vi "General Config.vi"(8 "error In":errorcluster, 10 "IOList":T2, 11 "reference":refnum<vi>) -> (0 "error out":errorcluster, 3 "Out reference":refnum<vi>)   [LabVIEW 2015]
uses:
  Control Button/Exit.ctl
  Control Button/Daq.ctl
  Control Button/Scanner config.ctl
  Control Button/Program Seq.ctl
  Control Button/cali.ctl
  Control Button/shift change.ctl
  Control Button/User mgt.ctl
  Control Button/model create.ctl
  Galobal variable_TI.vi
panel:
  in  "Image Setting":bool
  out "User Name 4":string
  in  "Load Cell Setting":bool
  out "User Name 3":string
  in  "Model Create":T1
  in  "User Mgt":T3
  out "User Name 2":string
  in  "Shift":T4
  in  "Calibration":T5
  in  "IO List Update":bool
  out "error out 2":errorcluster
  in  "error in (no error)":errorcluster
  in  "Program Seq":T6
  in  "Scanner config":T7
  in  "DAQ Config":T8
  out "User Name":string
  in  "Exit":T9
  out "String":string
  out "appended path":path
  in  "Ring":u16(ring)
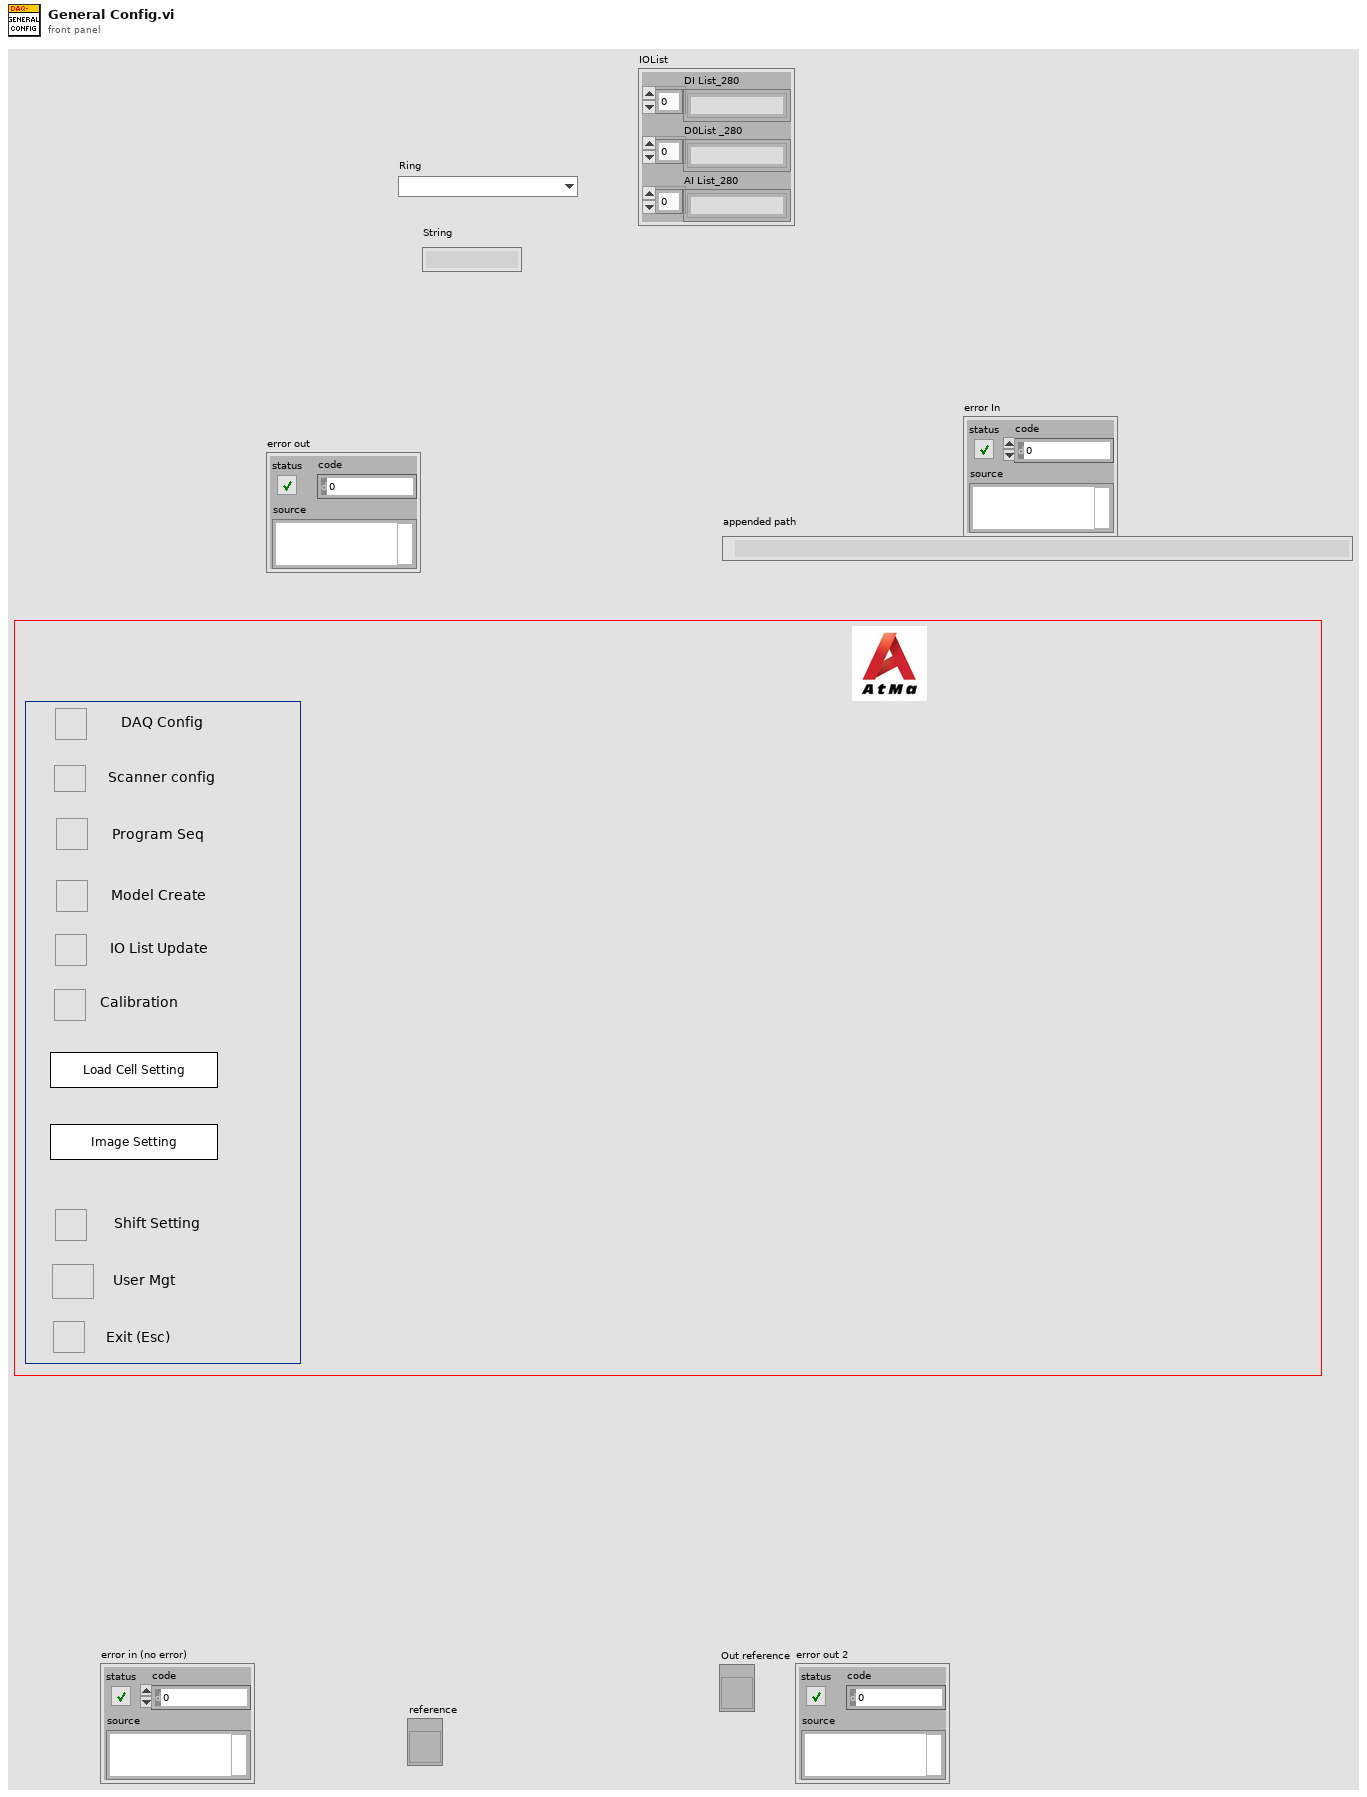
[diagram p1: front panel]
types:
  T1 = typedef "model create.ctl" = bool
  T2 = cluster{"DI List_280":string[], "D0List _280":string[], "AI List_280":string[]}
  T3 = typedef "User mgt.ctl" = bool
  T4 = typedef "shift change.ctl" = bool
  T5 = typedef "cali.ctl" = bool
  T6 = typedef "Program Seq.ctl" = bool
  T7 = typedef "Scanner config.ctl" = bool
  T8 = typedef "Daq.ctl" = bool
  T9 = typedef "Exit.ctl" = bool
  T10 = enum32{"Invalid", "Standard", "Closed", "Hidden", "Minimized", "Maximized"}
  T11 = cluster{"XInput":dbl[], "Y New Value":dbl[], "Avg point":i16}[]
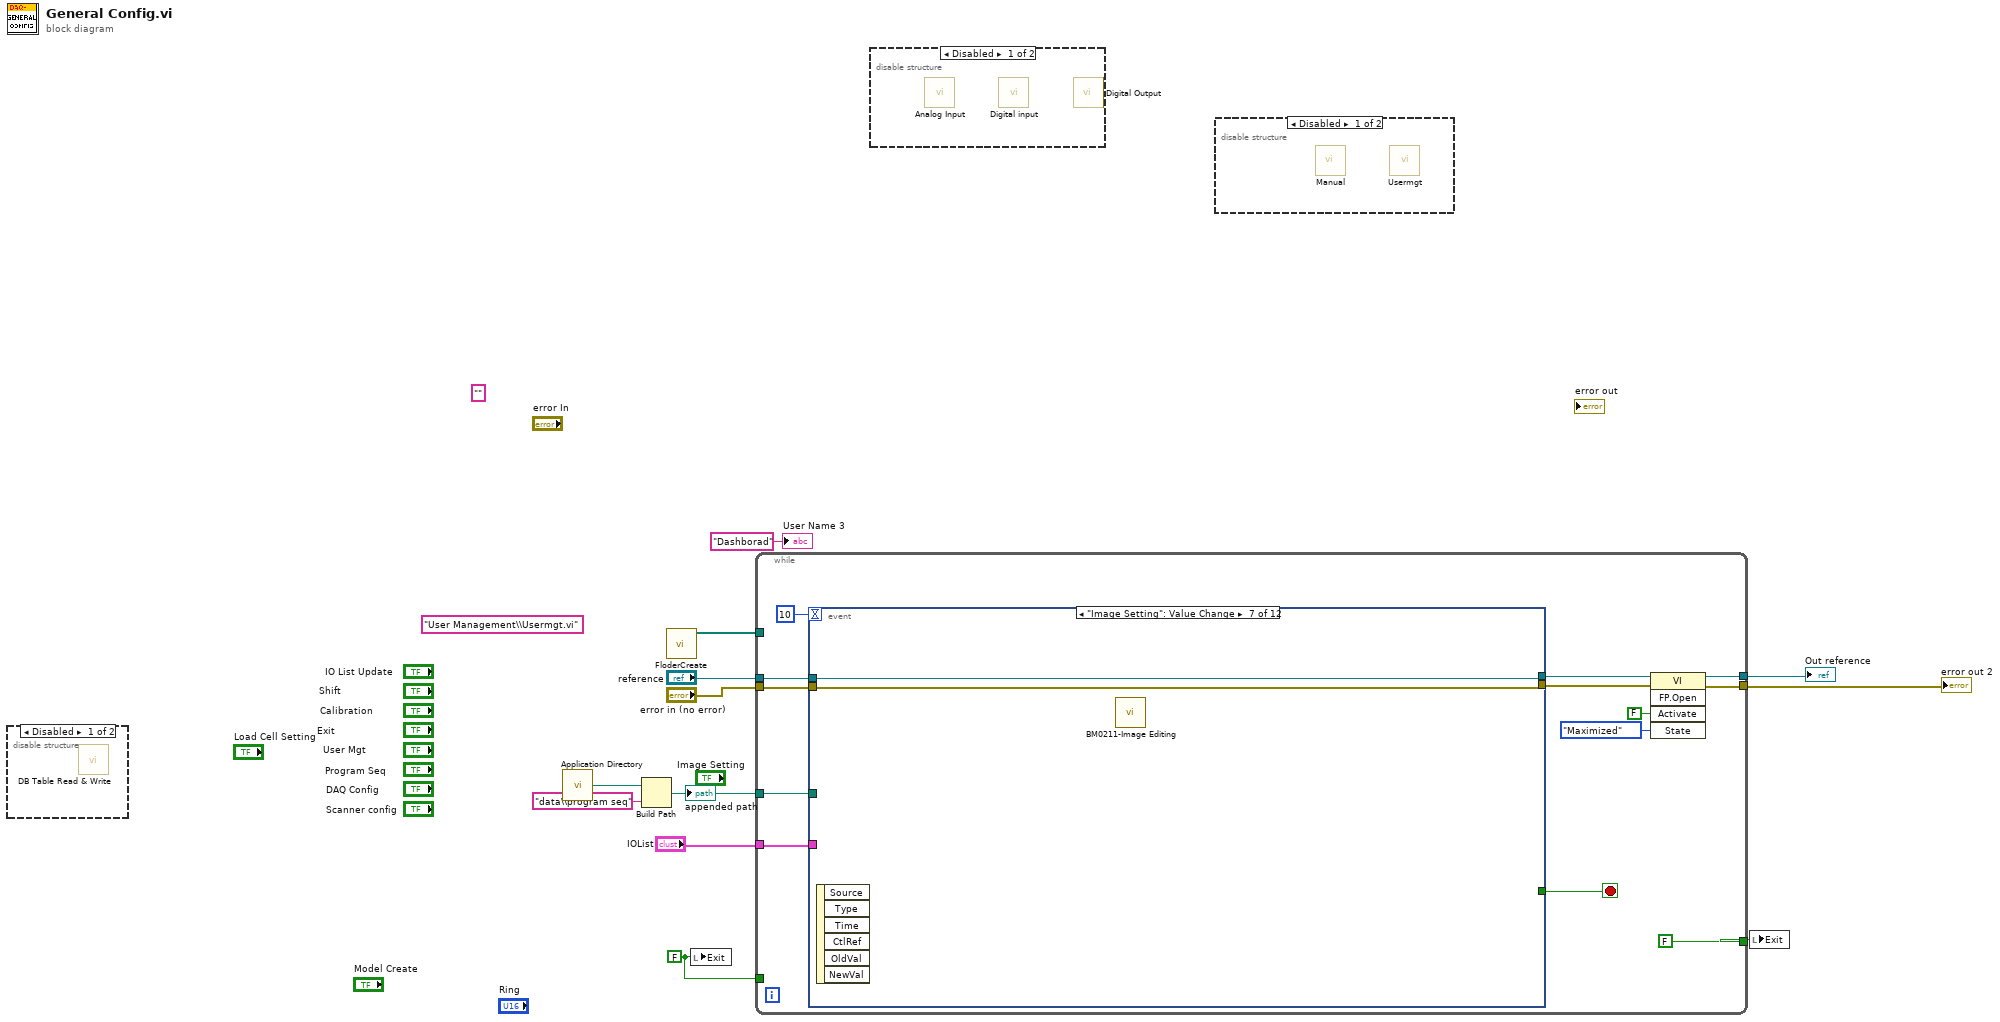
[diagram p0: block diagram]
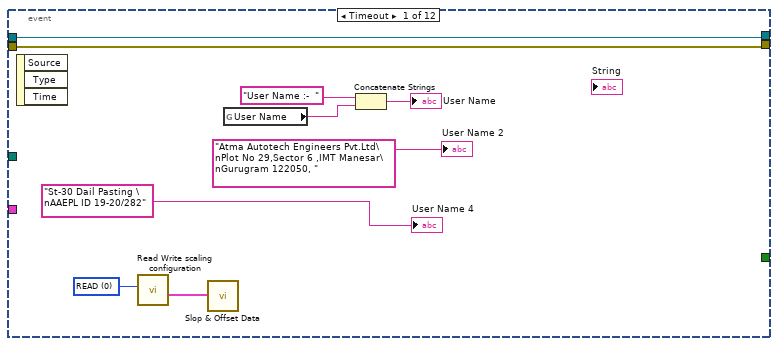
[diagram p5: hidden frame]
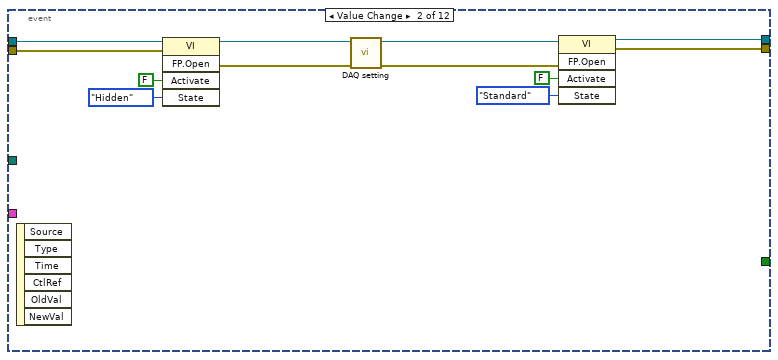
[diagram p6: hidden frame]
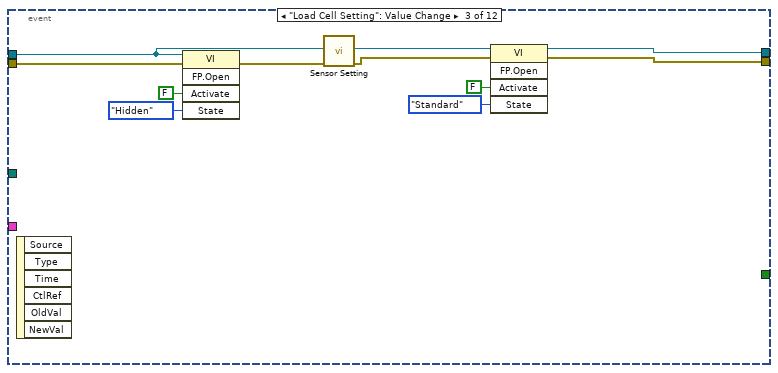
[diagram p7: hidden frame]
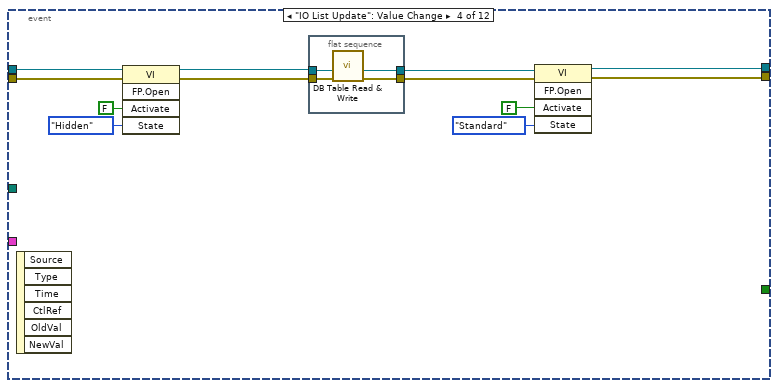
[diagram p8: hidden frame]
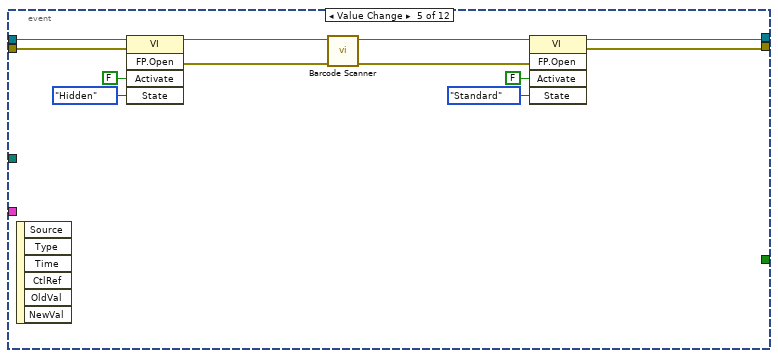
[diagram p9: hidden frame]
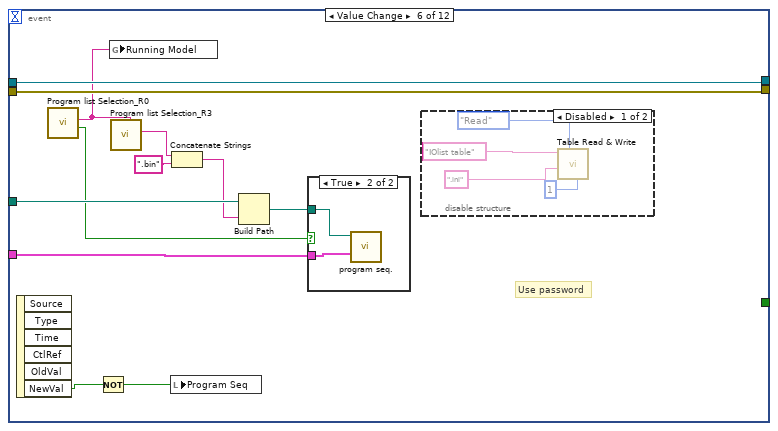
[diagram p10: hidden frame]
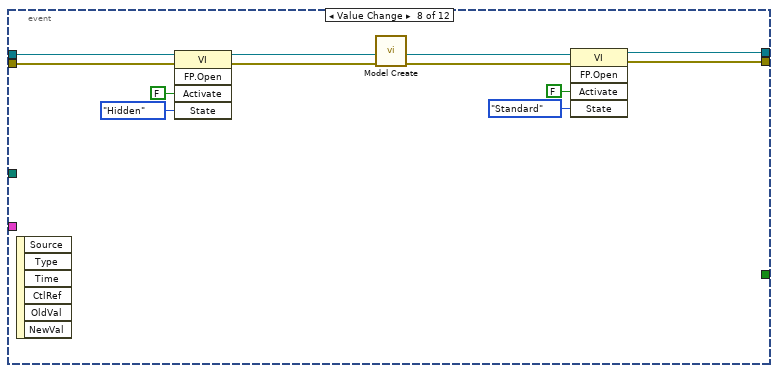
[diagram p13: hidden frame]
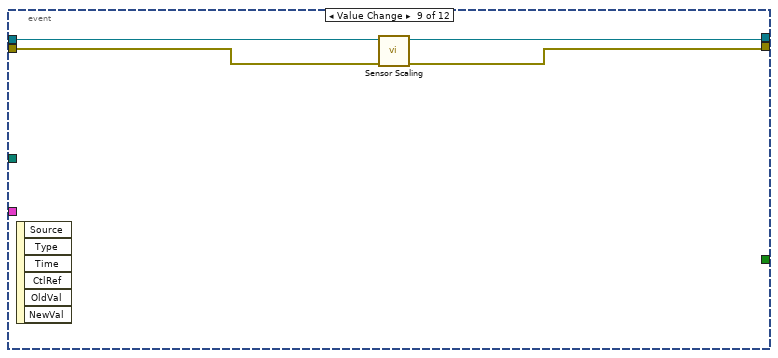
[diagram p14: hidden frame]
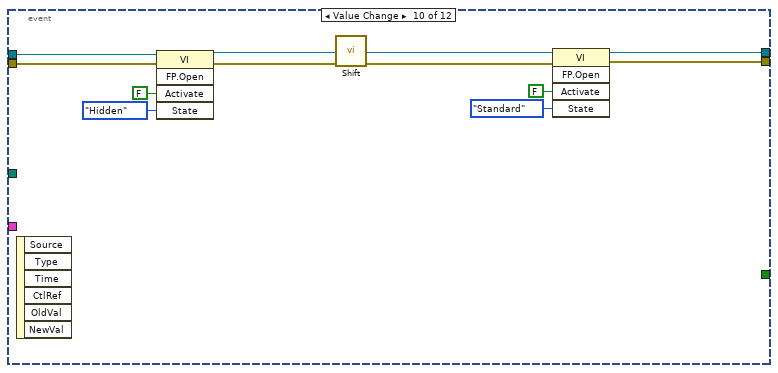
[diagram p15: hidden frame]
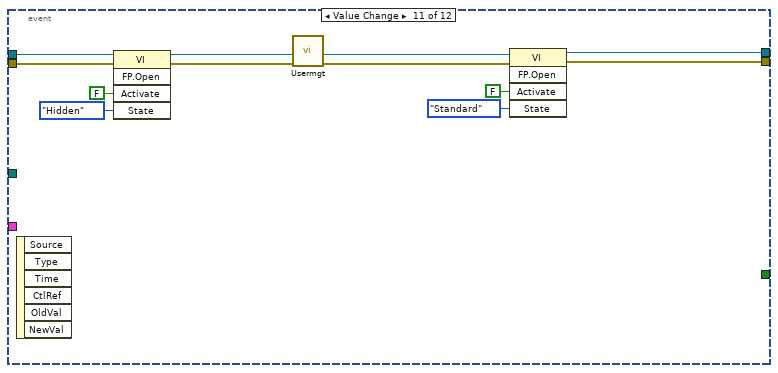
[diagram p16: hidden frame]
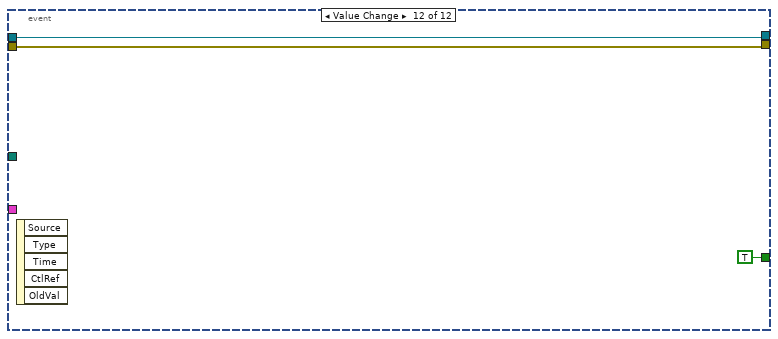
[diagram p17: hidden frame]
diagram:
  w9 = T9 FALSE ("Exit")
  (unwired) "User Management\\Usermgt.vi" ("name or relative path")
  (unwired) ""
  n1 = disable-structure shown="Disabled" {
    frame Disabled {
      n2 = call "DB Table Read & Write.vi"() -> ()  [unwired: 10 in, 2 out]
    }
    frame Enabled {
    }
  }
  n3 = call <vilib>:"Application Directory.vi"() -> ("Application Directory"=w5:path)
  n4 = Build Path(base path=w5, name or relative path="data\\program seq") -> (appended path=w2:path)
  "appended path" <- w2
  n5 = call "FloderCreate.vi"() -> ("File Path"=w6:path[])  [unwired: 11 in]
  n6 = local write "Exit"(w9) -> ()
  n7 = while {
    tunnel: w2 -> [w13]
    tunnel: "reference" -> [w23]
    tunnel: "error in (no error)" -> [w22]
    tunnel: [w17] -> w11
    tunnel: [w16] -> w10
    tunnel: w9 -> [_]
    tunnel: [T9 FALSE ("Exit")] -> w8
    tunnel: w6 -> [_]
    tunnel: "IOList" -> [w14]
    stop <- w24 stop-if-true
    n8 = event shown="[6] \"Image Setting\": Value Change" {
      selector: _ -> [_ _ _ _ _ _ _ _ _ _ _ _]
      dyn-events: _ -> [_ _ _ _ _ _ _ _ _ _ _ _]
      timeout: 10 -> [_ _ _ _ _ _ _ _ _ _ _ _]
      tunnel: [_ _ _ _ _ _ _ _ _ _ _ TRUE ("Exit")] -> w24
      tunnel: w23 -> [w31 w38 w48 w60 w82 w96 w104 w111 w118 w126 w135 w143]
      tunnel: w22 -> [w30 w37 w50 w59 w81 w95 w103 w110 w117 w124 w133 w142]
      tunnel: [w31 w36 w47 w67 w74 w96 w104 w106 w118 w125 w134 w143] -> w19
      tunnel: [w30 w35 w49 w66 w73 w95 w103 w105 w116 w123 w132 w142] -> w18
      tunnel: w14 -> [_ _ _ _ _ w94 _ _ _ _ _ _]
      tunnel: w13 -> [_ _ _ _ _ w93 _ _ _ _ _ _]
      event Timeout {
        w29 = u16 0 items=["READ", "WRITE"] ("Read/Write")
        n9 = event-data() -> ()  [unwired: 1 in, 3 out]
        n10 = call "Read Write scaling configuration.vi"("Read/Write"=w29) -> ("Output"=w28:T11)  [unwired: 4 in, 2 out]
        n11 = call "Slop & Offset Data.vi"("Input"=w28) -> ()  [unwired: 10 in, 1 out]
        n12 = global read "Galobal variable_TI.vi" "User Name"() -> (w34:string)
        n13 = Concatenate Strings("User Name :-  " ("string"), w34) -> (→"User Name":string)
        "User Name 2" <- "Atma Autotech Engineers Pvt.Ltd\nPlot No 29,Sector 6 ,IMT Manesar\nGurugram 122050, " ("string")
        "User Name 4" <- "St-30 Dail Pasting \nAAEPL ID 19-20/282" ("string")
      }
      event Value Change {
        n14 = event-data() -> ()  [unwired: 1 in, 6 out]
        n15 = invoke class="VI" method="FP.Open"(reference=w38, error in=w37, "Activate"=FALSE ("Activate?"), "State"=T10."Hidden") -> (reference out=w44:refnum<vi>, error out=w43:errorcluster)  [unwired: 1 in, 3 out]
        n16 = call "DAQ setting.vi"("error in (no error)"=w43, "vi reference"=w44) -> ("error Out"=w39:errorcluster, "Out reference"=w40:refnum<vi>)  [unwired: 8 in]
        n17 = invoke class="VI" method="FP.Open"(reference=w40, error in=w39, "Activate"=FALSE ("Activate?"), "State"=T10."Standard") -> (reference out=w36:refnum<vi>, error out=w35:errorcluster)  [unwired: 1 in, 3 out]
      }
      event "Load Cell Setting": Value Change {
        n18 = event-data() -> ()  [unwired: 1 in, 6 out]
        n19 = invoke class="VI" method="FP.Open"(reference=w48, error in=w50, "Activate"=FALSE ("Activate?"), "State"=T10."Hidden") -> (error out=w54:errorcluster)  [unwired: 1 in, 4 out]
        n20 = call "Sensor Setting.vi"("error in"=w54) -> ("error  out"=w51:errorcluster)  [unwired: 10 in]
        n21 = invoke class="VI" method="FP.Open"(reference=w48, error in=w51, "Activate"=FALSE ("Activate?"), "State"=T10."Standard") -> (reference out=w47:refnum<vi>, error out=w49:errorcluster)  [unwired: 1 in, 3 out]
      }
      event "IO List Update": Value Change {
        n22 = event-data() -> ()  [unwired: 1 in, 6 out]
        n23 = invoke class="VI" method="FP.Open"(reference=w60, error in=w59, "Activate"=FALSE ("Activate?"), "State"=T10."Hidden") -> (reference out=w58:refnum<vi>, error out=w57:errorcluster)  [unwired: 1 in, 3 out]
        n24 = flat-sequence {
          tunnel: [w69] -> w64
          tunnel: [w70] -> w63
          tunnel: w58 -> [w71]
          tunnel: w57 -> [w72]
          frame #0 {
            n25 = call "DB Table Read & Write.vi"("error in"=w72, "reference"=w71) -> ("error out"=w69:errorcluster, "referenceOut"=w70:refnum<vi>)  [unwired: 8 in]
          }
        }
        n26 = invoke class="VI" method="FP.Open"(reference=w63, error in=w64, "Activate"=FALSE ("Activate?"), "State"=T10."Standard") -> (reference out=w67:refnum<vi>, error out=w66:errorcluster)  [unwired: 1 in, 3 out]
      }
      event Value Change {
        n27 = event-data() -> ()  [unwired: 1 in, 6 out]
        n28 = invoke class="VI" method="FP.Open"(reference=w82, error in=w81, "Activate"=FALSE ("Activate?"), "State"=T10."Hidden") -> (reference out=w78:refnum<vi>, error out=w77:errorcluster)  [unwired: 1 in, 3 out]
        n29 = call "Barcode Scanner.vi"("error in (no error)"=w77, "reference"=w78) -> ("error in (no error) 2"=w75:errorcluster, "reference 2"=w76:refnum<vi>)  [unwired: 8 in]
        n30 = invoke class="VI" method="FP.Open"(reference=w76, error in=w75, "Activate"=FALSE ("Activate?"), "State"=T10."Standard") -> (reference out=w74:refnum<vi>, error out=w73:errorcluster)  [unwired: 1 in, 3 out]
      }
      event Value Change {
        # "Use password"
        n31 = event-data() -> ("NewVal"=w88:T6)  [unwired: 1 in, 5 out]
        n32 = call "Program list Selection_R0.vi"() -> ("Exit"=w89:bool, "String"=w85:string)  [unwired: 8 in, 2 out]
        n33 = Not(x=w88) -> (.not. x?=w87:T6)
        n34 = global write "Galobal variable_TI.vi" "Running Model"(w85) -> ()
        n35 = call "Program list Selection_R3.vi"("new element/subarray"=w85) -> ("String"=w86:string)  [unwired: 7 in, 3 out]
        n36 = local write "Program Seq"(w87) -> ()
        n37 = Concatenate Strings(w86, ".bin" ("string")) -> (w92:string)
        n38 = Build Path(base path=w93, name or relative path=w92) -> (appended path=w90:path)
        n39 = case shown="True" w89 {
          tunnel: w94 -> [_ w97]
          tunnel: w90 -> [_ w98]
          frame False {
          }
          frame True {
            n40 = call "program seq..vi"("IOList"=w97, "Filepath"=w98) -> ()  [unwired: 9 in, 1 out]
          }
        }
        n41 = disable-structure shown="Disabled" {
          frame Disabled {
            n42 = call "Table Read & Write.vi"("File Name"="IOlist table", "File type"=".ini", "Enum"=enum16{"Read", "Write"}."Read", "index"=1) -> ()  [unwired: 5 in, 2 out]
          }
          frame Enabled {
          }
        }
      }
      event "Image Setting": Value Change {
        n43 = event-data() -> ()  [unwired: 1 in, 6 out]
        n44 = call "BM0211-Image Editing.vi"() -> ()  [unwired: 11 in, 1 out]
      }
      event Value Change {
        n45 = event-data() -> ()  [unwired: 1 in, 6 out]
        n46 = invoke class="VI" method="FP.Open"(reference=w111, error in=w110, "Activate"=FALSE ("Activate?"), "State"=T10."Hidden") -> (reference out=w107:refnum<vi>, error out=w109:errorcluster)  [unwired: 1 in, 3 out]
        n47 = call "Model Create.vi"("error in (no error)"=w109) -> ("error out"=w108:errorcluster)  [unwired: 10 in]
        n48 = invoke class="VI" method="FP.Open"(reference=w107, error in=w108, "Activate"=FALSE ("Activate?"), "State"=T10."Standard") -> (reference out=w106:refnum<vi>, error out=w105:errorcluster)  [unwired: 1 in, 3 out]
      }
      event Value Change {
        n49 = event-data() -> ()  [unwired: 1 in, 6 out]
        n50 = call "Sensor Scaling.vi"("error in"=w117) -> ("error out"=w116:errorcluster)  [unwired: 9 in, 1 out]
      }
      event Value Change {
        n51 = event-data() -> ()  [unwired: 1 in, 6 out]
        n52 = invoke class="VI" method="FP.Open"(reference=w126, error in=w124, "Activate"=FALSE ("Activate?"), "State"=T10."Hidden") -> (reference out=w127:refnum<vi>, error out=w129:errorcluster)  [unwired: 1 in, 3 out]
        n53 = call "Shift.vi"("error in"=w129) -> ("error out"=w128:errorcluster)  [unwired: 10 in]
        n54 = invoke class="VI" method="FP.Open"(reference=w127, error in=w128, "Activate"=FALSE ("Activate?"), "State"=T10."Standard") -> (reference out=w125:refnum<vi>, error out=w123:errorcluster)  [unwired: 1 in, 3 out]
      }
      event Value Change {
        n55 = event-data() -> ()  [unwired: 1 in, 6 out]
        n56 = invoke class="VI" method="FP.Open"(reference=w135, error in=w133, "Activate"=FALSE ("Activate?"), "State"=T10."Hidden") -> (reference out=w136:refnum<vi>, error out=w131:errorcluster)  [unwired: 1 in, 3 out]
        n57 = call "Usermgt.vi"("error In"=w131) -> ("error out"=w130:errorcluster)  [unwired: 10 in]
        n58 = invoke class="VI" method="FP.Open"(reference=w136, error in=w130, "Activate"=FALSE ("Activate?"), "State"=T10."Standard") -> (reference out=w134:refnum<vi>, error out=w132:errorcluster)  [unwired: 1 in, 3 out]
      }
      event Value Change {
        n59 = event-data() -> ()  [unwired: 1 in, 5 out]
      }
    }
    n60 = invoke class="VI" method="FP.Open"(reference=w19, error in=w18, "Activate"=FALSE ("Activate?"), "State"=T10."Maximized") -> (reference out=w17:refnum<vi>, error out=w16:errorcluster)  [unwired: 1 in, 3 out]
  }
  "Out reference" <- w11
  "error out 2" <- w10
  n61 = disable-structure shown="Disabled" {
    frame Disabled {
      n62 = call "Analog Input.vi"() -> ()  [unwired: 10 in, 2 out]
      n63 = call "Digital input.vi"() -> ()  [unwired: 10 in, 2 out]
      n64 = call "Digital Output.vi"() -> ()  [unwired: 10 in, 2 out]
    }
    frame Enabled {
    }
  }
  n65 = disable-structure shown="Disabled" {
    frame Disabled {
      n66 = call "Manual.vi"() -> ()  [unwired: 10 in, 2 out]
      n67 = call "Usermgt.vi"() -> ()  [unwired: 11 in, 1 out]
    }
    frame Enabled {
    }
  }
  n68 = local write "Exit"(w8) -> ()
  "User Name 3" <- "Dashborad" ("User Name 3")
